vi "GetWeeksInfo.vi"(8 "error in (no error)":errorcluster, 11 "Data Value Reference in":refnum<data-value>) -> (0 "error out":errorcluster, 2 "Current Week":i16, 3 "Data Value Reference out":refnum<data-value>)   [LabVIEW 2017, in "DS_Lib.lvlib" / "SRReportParser.lvlib"]
uses:
  SRReportParser.lvlib
  Modules/Private Controls/Report Data Cluster.ctl
  Modules/Private Controls/Data Raw.ctl
  Modules/Data Operations.lvlib
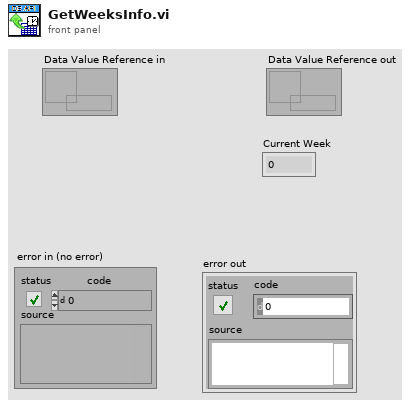
[diagram p1: front panel]
types:
  T1 = typedef "Data Operations.lvlib/Report Data Cluster.ctl" = cluster{"Headers":cluster{"Start Date":timestamp, "End Date":timestamp, "SR Status String":string[], "AE Owner String":string[]}, "Data":T2[]}
  T2 = typedef "Data Operations.lvlib/Data Raw.ctl" = cluster{"SR Number":string, "Status":string, "Summary":string, "AE Owner":string, "AE Group":string, "Contact":string, "SurveyData":cluster{"Resolution Time":dbl, "Total Satisfaction":dbl, "Response Time":dbl, "Courtesy":dbl, "Problem Solved":dbl, "Level of effort":dbl}, "Time Data":cluster{"Last Update Date":timestamp, "Creation Date":timestamp, "Creation week":i16, "Last Update Week":i16, "Creation Year":i16}}
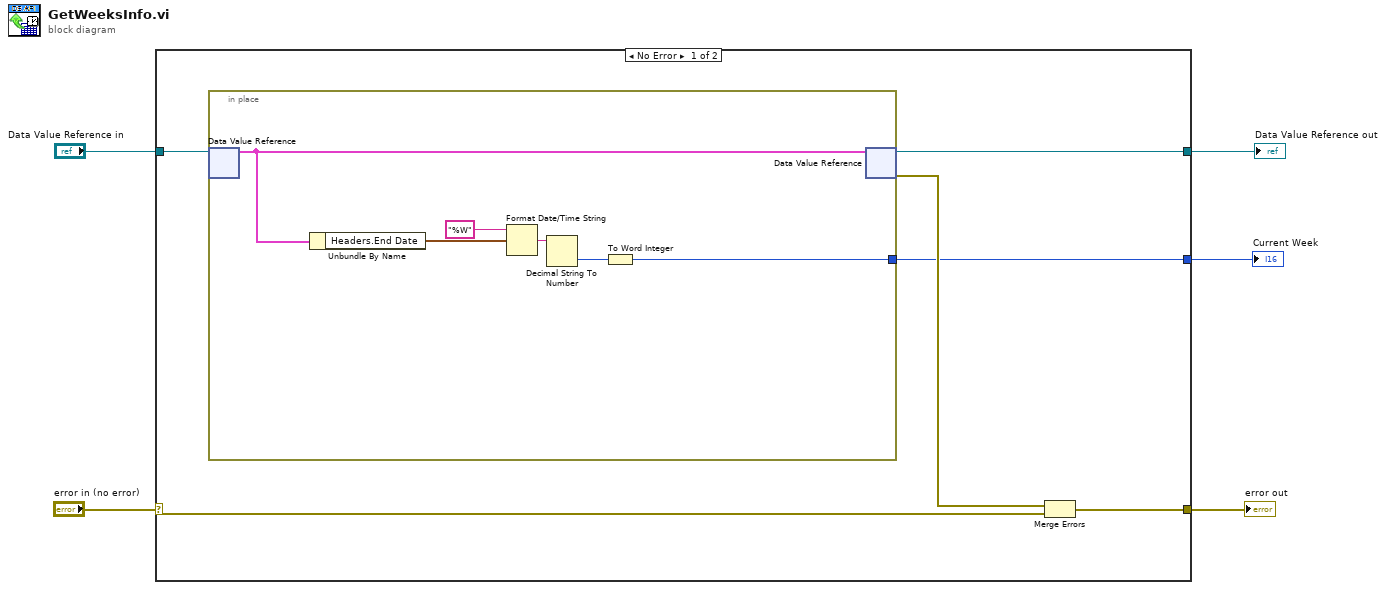
[diagram p0: block diagram]
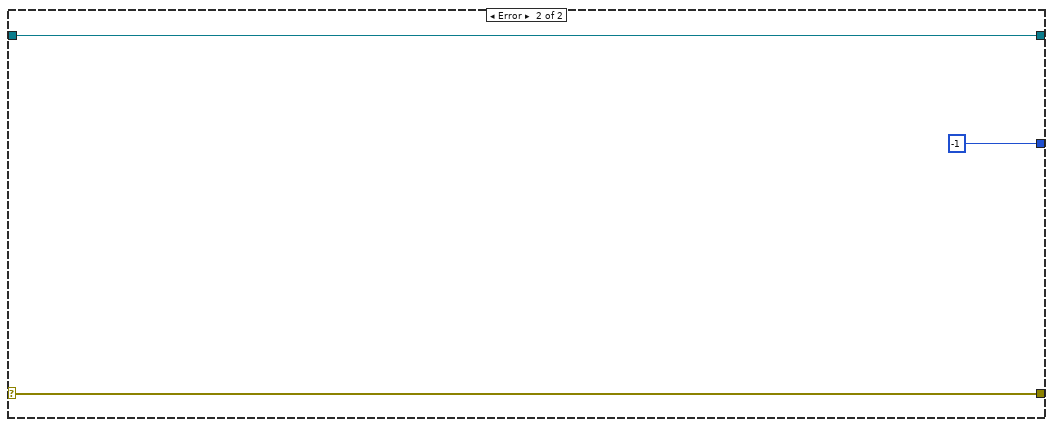
[diagram p2: hidden frame]
diagram:
  n1 = case shown="No Error" "error in (no error)" {
    selector: "error in (no error)" -> [w7 w20]
    tunnel: [w11 w19] -> w5
    tunnel: "Data Value Reference in" -> [w10 w19]
    tunnel: [w8 w20] -> w3
    tunnel: [w6 i16 -1] -> w1
    frame No Error {
      n2 = in-place {
        in-place-border: [w12] -> w6
        n3 = in-place-dvr #1(w10) -> (w17:T1)  [unwired: 1 out]
        n4 = Unbundle By Name(w17) -> ("Headers.End Date"=w15:timestamp)
        n5 = Format Date/Time String(time format string (%c)="%W", seconds (now)=w15) -> (date/time string=w16:string)  [unwired: 1 in]
        n6 = Decimal String To Number(string=w16) -> (number=w13:i32)  [unwired: 2 in, 1 out]
        n7 = To Word Integer(number=w13) -> (16bit integer=w12:i16)
        n8 = in-place-dvr #1(w17) -> (w11:refnum<data-value>, w9:errorcluster)
      }
      n9 = Merge Errors(w9, w7) -> (w8:errorcluster)
    }
    frame Error {
    }
  }
  "error out" <- w3
  "Data Value Reference out" <- w5
  "Current Week" <- w1
